vi "2-5.vi"() -> ()   [LabVIEW 2018]
panel:
  in  "选项卡控件":enum32{"2-1", "2-2", "2-3", "2-4"}(tab)
  in  "停止":bool
  out "时域":waveform(dbl)[](graph)
  in  "载波信号":cluster{"fc(Hz)":dbl, "Ac(V)":dbl}={"fc(Hz)"=150000.0, "Ac(V)"=1.0}
  in  "调制信号":cluster{"fm(Hz)":dbl, "Am(V)":dbl}={"fm(Hz)"=5000.0, "Am(V)"=1.0}
  in  "An(V)":dbl=0.02
  in  "kf(Hz/V)":dbl=50000.0
  in  "带通Butterworth滤波器":cluster{"中心频率(Hz)":dbl, "带宽(Hz)":dbl}={"中心频率(Hz)"=150000.0, "带宽(Hz)"=220000.0}
  in  "开始":bool
  out "时域 2":waveform(dbl)[](graph)
  out "频域":cluster{"f0":dbl, "df":dbl, "magnitude":dbl[]}(graph)
  in  "开始 2":bool
  in  "停止 2":bool
  in  "载波信号 2":cluster{"fc(Hz)":dbl, "Ac(V)":dbl}={"fc(Hz)"=150000.0, "Ac(V)"=1.0}
  in  "调制信号 2":T1={"fm1(Hz)"=5000.0, "Am(V)"=1.0, "fm2(Hz)"=3000.0}
  in  "An(V) 2":dbl=0.1
  in  "kf(Hz/V) 2":dbl=50000.0
  in  "带通Butterworth滤波器 2":cluster{"中心频率(Hz)":dbl, "带宽(Hz)":dbl}={"中心频率(Hz)"=150000.0, "带宽(Hz)"=280000.0}
  out "频域 2":cluster{"f0":dbl, "df":dbl, "magnitude":dbl[]}(graph)
  out "时域 4":waveform(dbl)[](graph)
  out "时域 3":waveform(dbl)[](graph)
  in  "停止 3":bool
  in  "开始 3":bool
  in  "载波信号 3":cluster{"fc(Hz)":dbl, "Ac(V)":dbl}={"fc(Hz)"=150000.0, "Ac(V)"=1.0}
  in  "调制信号 3":cluster{"T(s)":dbl, "Am(V)":dbl}={"T(s)"=0.0002, "Am(V)"=1.0}
  in  "An(V) 3":dbl=0.1
  in  "kf(Hz/V) 3":dbl=50000.0
  in  "带通Butterworth滤波器 3":cluster{"中心频率(Hz)":dbl, "带宽(Hz)":dbl}={"中心频率(Hz)"=150000.0, "带宽(Hz)"=280000.0}
  out "频域 3":cluster{"f0":dbl, "df":dbl, "magnitude":dbl[]}(graph)
  out "时域 6":waveform(dbl)[](graph)
  out "时域 5":waveform(dbl)[](graph)
  in  "停止 4":bool
  in  "开始 4":bool
  in  "载波信号 4":cluster{"fc(Hz)":dbl, "Ac(V)":dbl}={"fc(Hz)"=150000.0, "Ac(V)"=1.0}
  in  "调制信号 4":cluster{"T(s)":dbl, "Am(V)":dbl}={"T(s)"=0.0002, "Am(V)"=1.0}
  in  "An(V) 4":dbl=0.1
  in  "kf(Hz/V) 4":dbl=50000.0
  in  "带通Butterworth滤波器 4":cluster{"中心频率(Hz)":dbl, "带宽(Hz)":dbl}={"中心频率(Hz)"=150000.0, "带宽(Hz)"=220000.0}
  out "时域 7":waveform(dbl)[](graph)
  out "时域 8":waveform(dbl)[](graph)
  out "频域 4":cluster{"f0":dbl, "df":dbl, "magnitude":dbl[]}(graph)
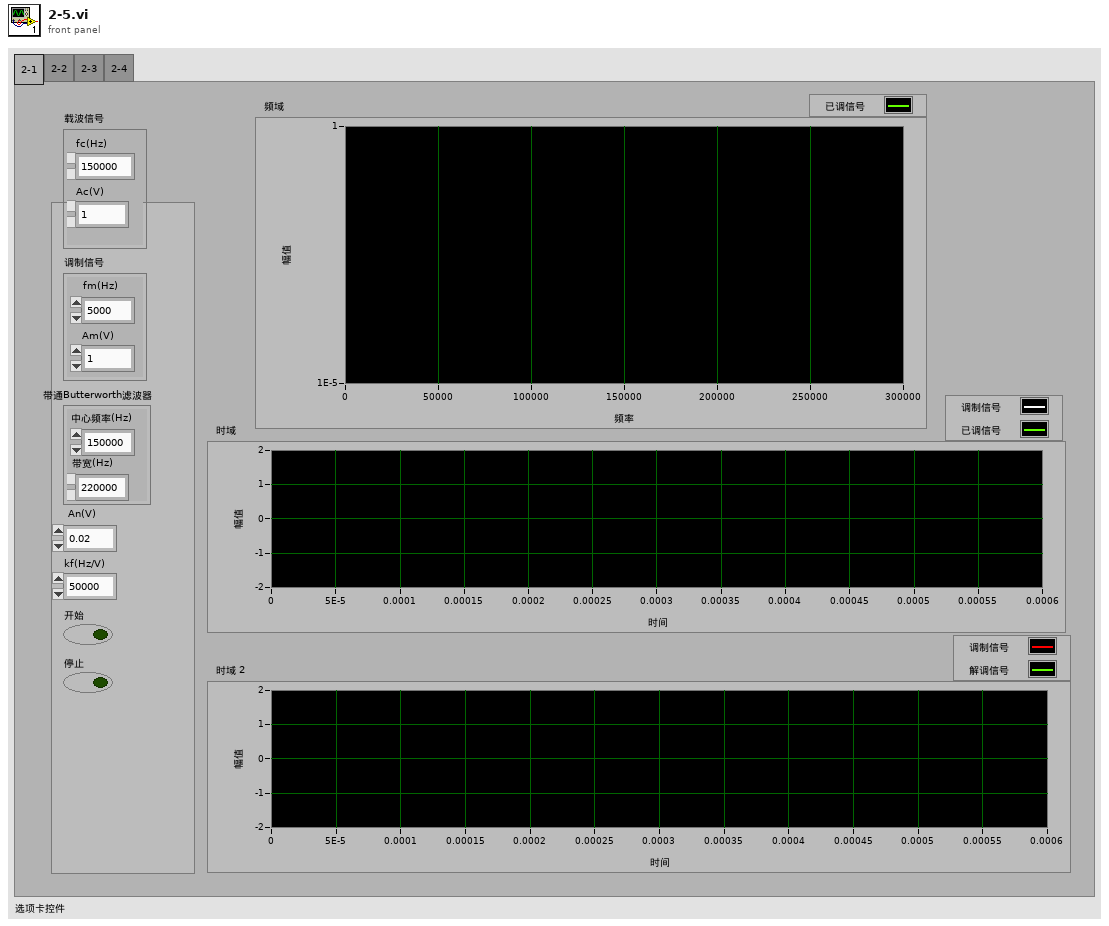
[diagram p1: front panel]
types:
  T1 = cluster{"fm1(Hz)":dbl, "Am(V)":dbl, "fm2(Hz)":dbl}
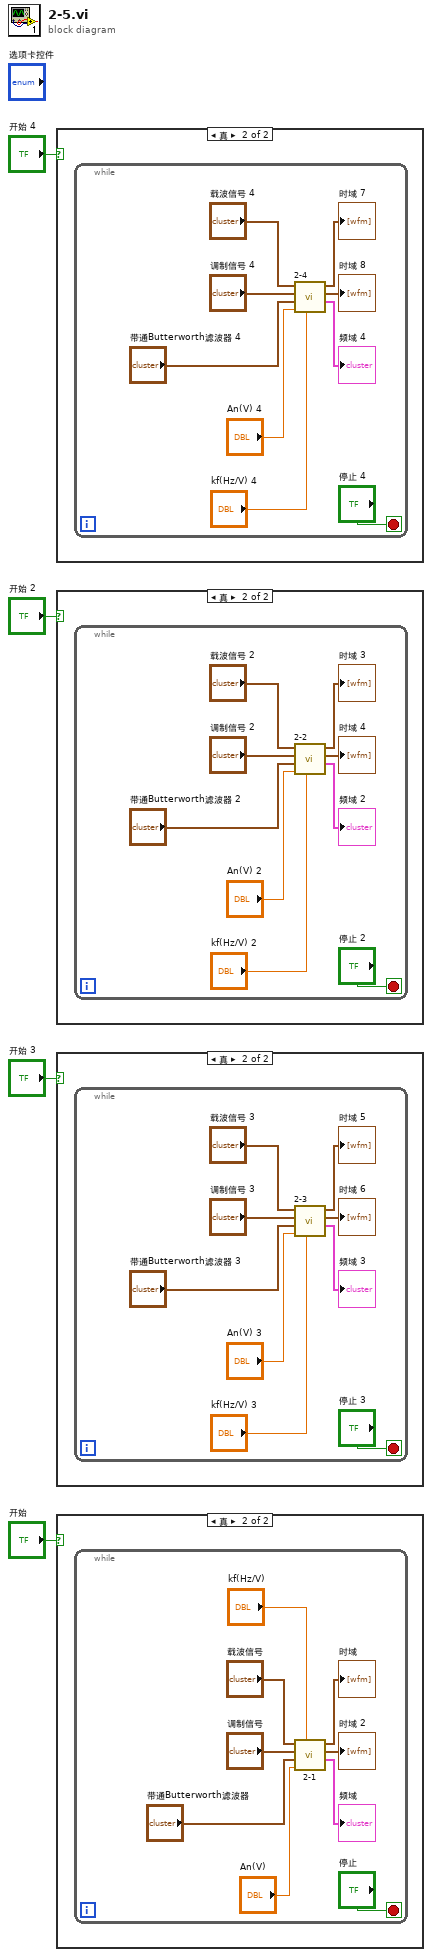
[diagram p0: block diagram]
diagram:
  n1 = case shown="真" "开始 4" {
    frame False {
    }
    frame True {
      n2 = while {
        stop <- "停止 4" stop-if-true
        n3 = call "2-4.vi"("kf(Hz/V)"="kf(Hz/V) 4", "An(V)"="An(V) 4", "带通Butterworth滤波器"="带通Butterworth滤波器 4", "调制信号"="调制信号 4", "载波信号"="载波信号 4") -> ("频域"=→"频域 4":cluster{"f0":dbl, "df":dbl, "magnitude":dbl[]}, "时域 2"=→"时域 8":waveform(dbl)[], "时域"=→"时域 7":waveform(dbl)[])  [unwired: 4 in]
      }
    }
  }
  n4 = case shown="真" "开始 2" {
    frame False {
    }
    frame True {
      n5 = while {
        stop <- "停止 2" stop-if-true
        n6 = call "2-2.vi"("kf(Hz/V)"="kf(Hz/V) 2", "An(V)"="An(V) 2", "带通Butterworth滤波器"="带通Butterworth滤波器 2", "调制信号"="调制信号 2", "载波信号"="载波信号 2") -> ("频域"=→"频域 2":cluster{"f0":dbl, "df":dbl, "magnitude":dbl[]}, "时域 2"=→"时域 4":waveform(dbl)[], "时域"=→"时域 3":waveform(dbl)[])  [unwired: 4 in]
      }
    }
  }
  n7 = case shown="真" "开始 3" {
    frame False {
    }
    frame True {
      n8 = while {
        stop <- "停止 3" stop-if-true
        n9 = call "2-3.vi"("kf(Hz/V)"="kf(Hz/V) 3", "An(V)"="An(V) 3", "带通Butterworth滤波器"="带通Butterworth滤波器 3", "调制信号"="调制信号 3", "载波信号"="载波信号 3") -> ("频域"=→"频域 3":cluster{"f0":dbl, "df":dbl, "magnitude":dbl[]}, "时域 2"=→"时域 6":waveform(dbl)[], "时域"=→"时域 5":waveform(dbl)[])  [unwired: 4 in]
      }
    }
  }
  n10 = case shown="真" "开始" {
    frame False {
    }
    frame True {
      n11 = while {
        stop <- "停止" stop-if-true
        n12 = call "2-1.vi"("kf(Hz/V)"="kf(Hz/V)", "An(V)"="An(V)", "带通Butterworth滤波器"="带通Butterworth滤波器", "调制信号"="调制信号", "载波信号"="载波信号") -> ("频域"=→"频域":cluster{"f0":dbl, "df":dbl, "magnitude":dbl[]}, "时域 2"=→"时域 2":waveform(dbl)[], "时域"=→"时域":waveform(dbl)[])  [unwired: 4 in]
      }
    }
  }
